vi "rqcBob ServiceNET Read Command.vi"(8 "error in":errorcluster, 11 "rqcBob ServiceNET in":T2) -> (0 "error out":errorcluster, 1 "cmd valid":bool, 2 "command":T1=enum."READY", 3 "rqcBob ServiceNET out":T2)   [LabVIEW 2018]
uses:
  Custom Controls/rqcBob ServiceNET control.ctl
  Custom Controls/rqc ServiceNET command.ctl
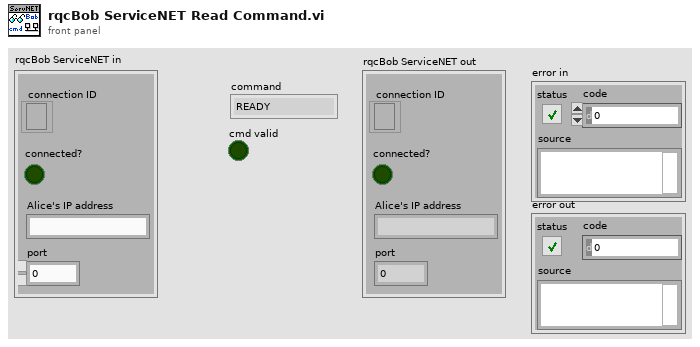
[diagram p1: front panel]
types:
  T1 = typedef "rqc ServiceNET command.ctl" = enum8{"NONE", "READY", "START", "PING"}
  T2 = typedef "rqcBob ServiceNET control.ctl" = cluster{"connection ID":refnum<k5>, "connected?":bool, "Alice's IP address":string, "port":u16}
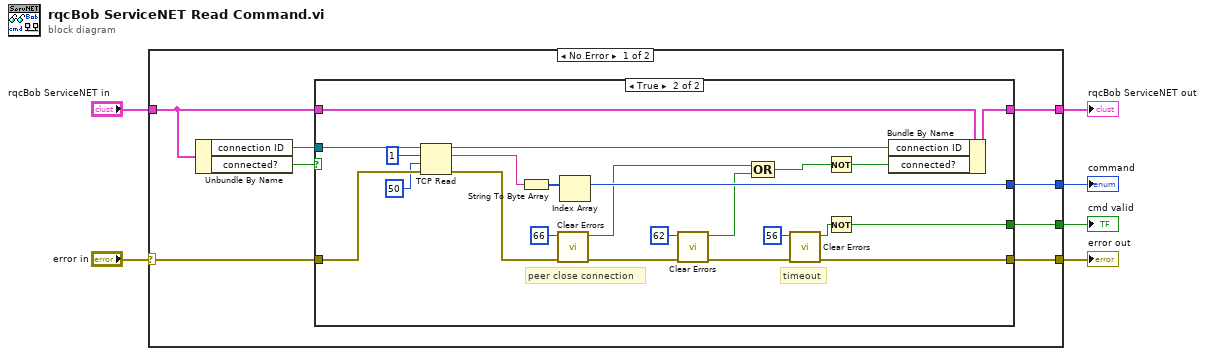
[diagram p0: block diagram]
diagram:
  n1 = case shown="No Error" "error in" {
    selector: "error in" -> [w12 w41]
    tunnel: "rqcBob ServiceNET in" -> [w10 w40]
    tunnel: [w11 w41] -> w4
    tunnel: [w9 w40] -> w3
    tunnel: [w8 _] -> w2
    tunnel: [w7 _] -> w1
    frame No Error {
      n2 = Unbundle By Name(w10) -> ("connection ID"=w13:refnum<k5>, "connected?"=w14:bool)
      n3 = case shown="True" w14 {
        tunnel: w13 -> [_ w37]
        tunnel: w12 -> [w16 w35]
        tunnel: [w16 w26] -> w11
        tunnel: [w15 w38] -> w9
        tunnel: w10 -> [w15 w39]
        tunnel: [_ w31] -> w8
        tunnel: [_ w23] -> w7
        frame False {
        }
        frame True {
          # "peer close connection"
          # "timeout"
          n4 = TCP Read(connection ID=w37, bytes to read=1, error in (no error)=w35, 9:50 ("timeout ms (25000)")) -> (connection ID out=w36:refnum<k5>, data out=w33:string, error out=w25:errorcluster)  [unwired: 1 in]
          n5 = String To Byte Array(string=w33) -> (unsigned byte array=w32:u8[])
          n6 = call <vilib>:"Clear Errors.vi"("error in (no error)"=w25, "specific error code to clear (0: all)"=66) -> ("error out"=w22:errorcluster, "specific error cleared?"=w19:bool)  [unwired: 4 in]
          n7 = Index Array(array=w32) -> (element=w31:u8)  [unwired: 1 in]
          n8 = call <vilib>:"Clear Errors.vi"("error in (no error)"=w22, "specific error code to clear (0: all)"=62) -> ("error out"=w21:errorcluster, "specific error cleared?"=w17:bool)  [unwired: 4 in]
          n9 = Compound Arithmetic op=OR(w19, w17) -> (w18:bool)
          n10 = call <vilib>:"Clear Errors.vi"("error in (no error)"=w21, "specific error code to clear (0: all)"=56) -> ("error out"=w26:errorcluster, "specific error cleared?"=w24:bool)  [unwired: 4 in]
          n11 = Not(x=w18) -> (.not. x?=w27:bool)
          n12 = Not(x=w24) -> (.not. x?=w23:bool)
          n13 = Bundle By Name(cluster=w39, "connection ID"=w36, "connected?"=w27) -> (w38:T2)
        }
      }
    }
    frame Error {
    }
  }
  "error out" <- w4
  "rqcBob ServiceNET out" <- w3
  "command" <- w2
  "cmd valid" <- w1
